vi "Get Row Tag.vi"(8 "error in":errorcluster, 10 "Row Index":i32, 11 "SourceGrid in":refnum<class "SourceGrid.lvclass">) -> (0 "error out":errorcluster, 2 "object":variant, 3 "SourceGrid out":refnum<class "SourceGrid.lvclass">)   [LabVIEW 2023, in "SourceGrid.lvlib" / "SourceGrid.lvclass"]
uses:
  SourceGrid.lvclass
  SourceGrid.lvclass/SourceGrid.ctl
  D:/git/Sourcegrid-LabVIEW/dll/SourceGrid.dll
  dll/SourceGrid.dll
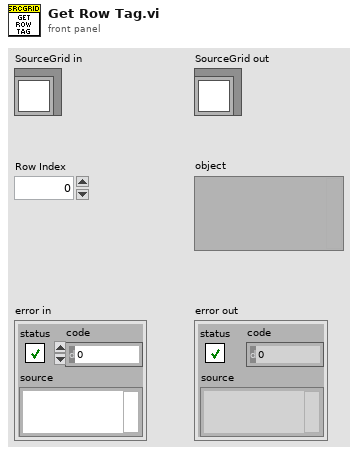
[diagram p1: front panel]
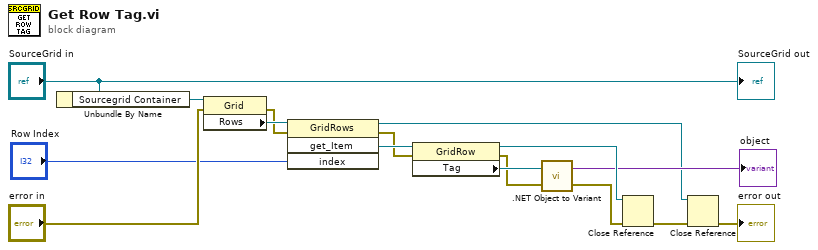
[diagram p0: block diagram]
diagram:
  n1 = Unbundle By Name("SourceGrid in") -> ("Sourcegrid Container"=w11:refnum<k24>)
  n2 = property class="Grid"(reference=w11, error in="error in") -> (error out=w13:errorcluster, "Rows"=w15:refnum<k24>)  [unwired: 1 out]
  n3 = invoke class="GridRows" method="get_Item"(reference=w15, error in=w13, "index"="Row Index") -> (reference out=w1:refnum<k24>, error out=w12:errorcluster, "get_Item"=w14:refnum<k24>)  [unwired: 1 in, 1 out]
  n4 = property class="GridRow"(reference=w14, error in=w12) -> (reference out=w7:refnum<k24>, error out=w5:errorcluster, "Tag"=w6:refnum<k24>)
  n5 = call <vilib>:".NET Object to Variant.vi"("error in (no error)"=w5, ".NET object"=w6) -> ("error out"=w4:errorcluster, "variant"=→"object":variant)
  n6 = Close Reference(reference=w7, error in (no error)=w4) -> (error out=w8:errorcluster)
  n7 = Close Reference(reference=w1, error in (no error)=w8) -> (error out=→"error out":errorcluster)
  "SourceGrid out" <- "SourceGrid in"
